vi "PositionToReceivePass3rdStriker.vi"(8 "error in (no error)":errorcluster, 9 "Robot":refnum<class "Robot.lvclass">, 10 "Game":refnum<class "Game.lvclass">, 11 "PositionToReceivePassSkill in":refnum<class "PositionToReceivePassSkill.lvclass">) -> (0 "error out":errorcluster, 2 "3rdStrikerPosition":dbl[](array[numeric]), 3 "PositionToReceivePassSkill out":refnum<class "PositionToReceivePassSkill.lvclass">)   [LabVIEW 2020, in "PositionToReceivePassSkill.lvclass"]
uses:
  PositionToReceivePassSkill.lvclass
  Game_class/Game.lvclass
  Robot_class/Robot.lvclass
  Game_class/Game.lvclass/Game.ctl
  Object_class/Object.lvclass/Object.ctl
  Game_class/Read BallRef.vi
  Object_class/Read x.vi
  Object_class/Read y.vi
  Ball_class/Ball.lvclass
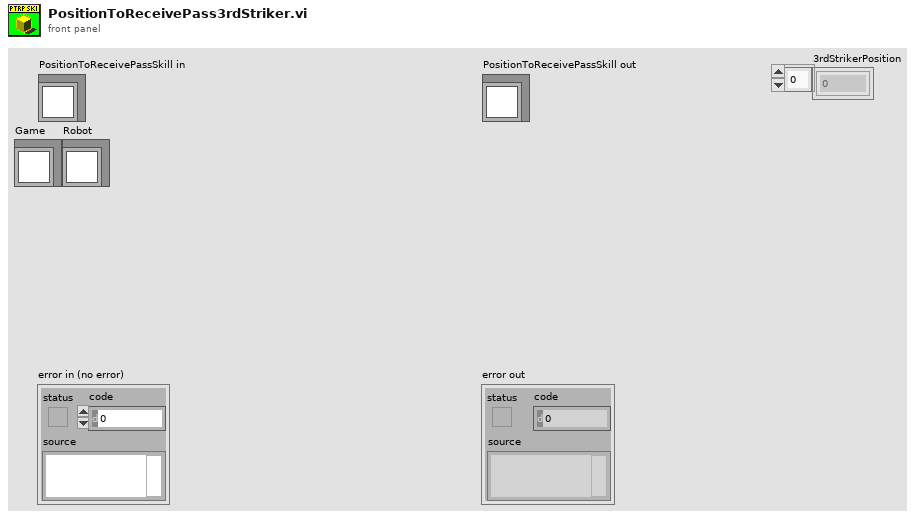
[diagram p1: front panel]
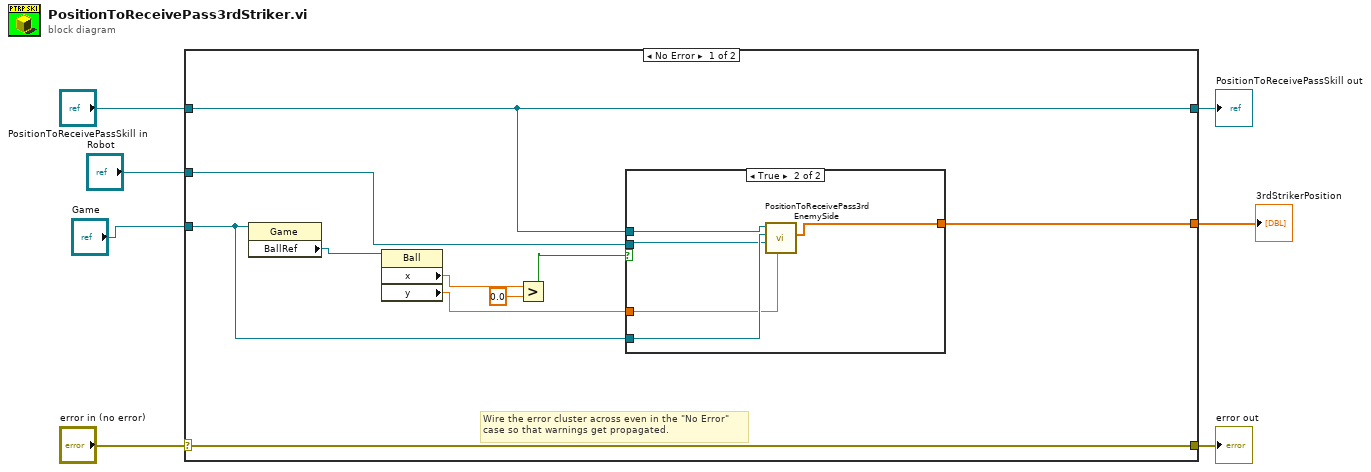
[diagram p0: block diagram]
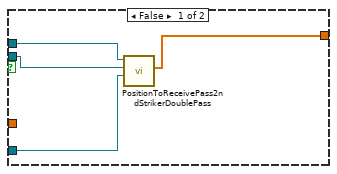
[diagram p2: hidden frame]
diagram:
  n1 = case shown="No Error" "error in (no error)" {
    selector: "error in (no error)" -> [w17 w28]
    tunnel: [w17 w28] -> w6
    tunnel: [w11 w27] -> w4
    tunnel: "PositionToReceivePassSkill in" -> [w11 w27]
    tunnel: "Game" -> [w12 _]
    tunnel: "Robot" -> [w10 _]
    tunnel: [w9 _] -> w1
    frame No Error {
      # "Wire the error cluster across even in the \"No Error\"\ncase so that warnings get propagated."
      n2 = property class="Game"(reference=w12) -> ("BallRef"=w16:refnum<class "Ball.lvclass">)  [unwired: 1 in, 2 out]
      n3 = property class="Ball"(reference=w16) -> ("x"=w15:dbl, "y"=w8:dbl)  [unwired: 1 in, 2 out]
      n4 = Greater?(x=w15, y=0.0) -> (0:w13:bool)
      n5 = case shown="True" w13 {
        tunnel: w12 -> [w21 w25]
        tunnel: w11 -> [w20 w26]
        tunnel: w10 -> [w19 w24]
        tunnel: [w18 w23] -> w9
        tunnel: w8 -> [_ w22]
        frame False {
          n6 = call "PositionToReceivePass2ndStrikerDoublePass.vi"("Game"=w21, "Robot"=w19, "PositionToReceivePassSkill in"=w20) -> ("2ndStrikerPositionDoublePass"=w18:dbl[])  [unwired: 6 in, 2 out]
        }
        frame True {
          n7 = call-dynamic "PositionToReceivePass3rdEnemySide.vi"("y ball"=w22, "Robot"=w24, "Game"=w25, "PositionToReceivePassSkill in"=w26) -> ("3rdStrikerPosition"=w23:dbl[])  [unwired: 5 in, 2 out]
        }
      }
    }
    frame Error {
    }
  }
  "error out" <- w6
  "PositionToReceivePassSkill out" <- w4
  "3rdStrikerPosition" <- w1
